vi "Helper SubVI - Get Single-level Coefficients and Reconstructions.vi"(5 "type":enum16{"Apprx", "Detail"}(ring), 6 "synthesis filters":cluster{"lowpass":dbl[], "highpass":dbl[]} {"highpass" format="%.2f"; "lowpass" format="%.2f"}, 7 "level":i32, 8 "error in (no error)":errorcluster, 9 "wavelet":u16(ring) items=["db02"=0, "db03"=1, "db04"=2, "db05"=3, "db06"=4, "db07"=5, "db08"=6, "db09"=7, "db10"=8, "db11"=9, "db12"=10, "db13"=11, "db14"=12, "Haar"=13, "bior1_3"=14, "bior1_5"=15, "bior2_2"=16, "bior2_4"=17, "bior2_6"=18, "bior2_8"=19, "bior3_1"=20, "bior3_3"=21, "bior3_5"=22, "bior3_7"=23, "bior3_9"=24, "bior4_4 (FBI)"=25, "bior5_5"=38, "bior6_8"=39, "coif1"=26, "coif2"=27, "coif3"=28, "coif4"=29, "coif5"=30, "sym2"=31, "sym3"=32, "sym4"=33, "sym5"=34, "sym6"=35, "sym7"=36, "sym8"=37], 10 "Lengths":i32[](array[numeric]), 11 "DWT":dbl[](array[numeric]) format="%.2f") -> (0 "error out":errorcluster, 2 "Reconstruction":dbl[](array[numeric]), 3 "Coeffs":dbl[](array[numeric]) format="%.2f")   [LabVIEW 2023]
doc: "Gets single-level coefficients and returns the reconstructed signal."
uses:
  <vilib>/addons/Wavelet Analysis/discrete wavelet transform.llb/WA Inverse 1D Discrete Wavelet Transform (Array).vi
  <vilib>/addons/_Advanced Signal Processing/NI_AdvSigProcWA.lvlib
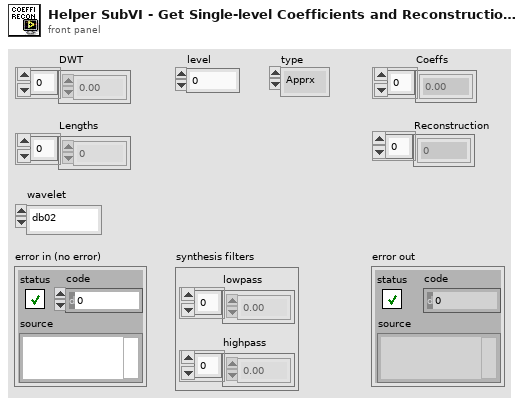
[diagram p1: front panel]
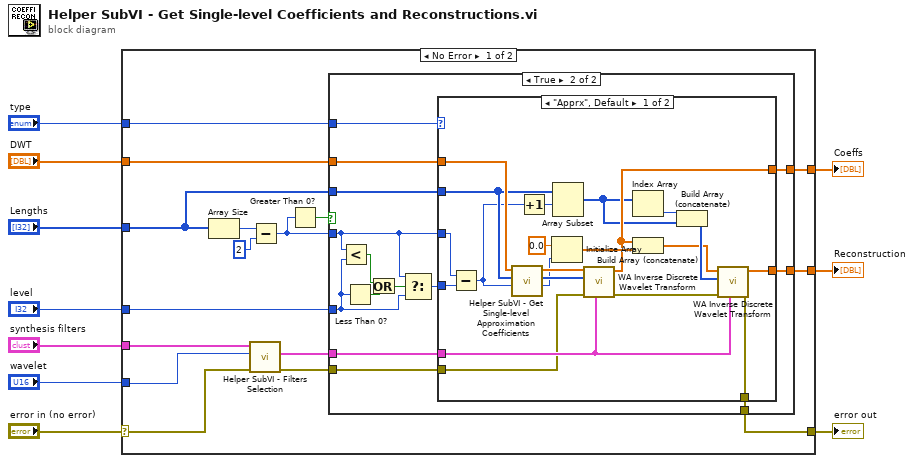
[diagram p0: block diagram]
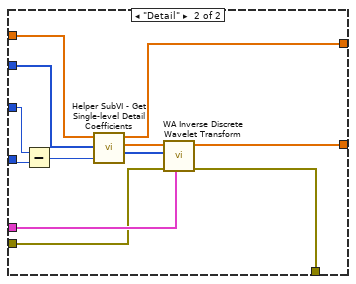
[diagram p3: hidden frame]
diagram:
  n1 = case shown="No Error" "error in (no error)" {
    selector: "error in (no error)" -> [w11 w75]
    tunnel: [w22 w75] -> w9
    tunnel: "DWT" -> [w21 _]
    tunnel: "Lengths" -> [w20 _]
    tunnel: "level" -> [w19 _]
    tunnel: "synthesis filters" -> [w18 _]
    tunnel: "wavelet" -> [w15 _]
    tunnel: [w17 _] -> w3
    tunnel: [w16 _] -> w2
    tunnel: "type" -> [w13 _]
    frame No Error {
      n2 = Array Size(array=w20) -> (size(s)=w26:i32)
      n3 = call "Helper SubVI - Filters Selection.vi"("error in (no error)"=w11, "wavelet"=w15, "filters"=w18) -> ("error out"=w12:errorcluster, "synthesis filters"=w14:cluster{"lowpass":dbl[], "highpass":dbl[]})  [unwired: 6 in, 1 out]
      n4 = Subtract(x=w26, y=2) -> (x-y=w23:i32)
      n5 = Greater Than 0?(x=w23) -> (x > 0?=w24:bool)
      n6 = case shown="True" w24 {
        tunnel: w21 -> [_ w39]
        tunnel: [_ w40] -> w16
        tunnel: w23 -> [_ w32]
        tunnel: w19 -> [_ w31]
        tunnel: w20 -> [_ w41]
        tunnel: w14 -> [_ w38]
        tunnel: [w27 w37] -> w22
        tunnel: [_ w36] -> w17
        tunnel: w13 -> [_ w29]
        tunnel: w12 -> [w27 w28]
        frame False {
        }
        frame True {
          n7 = Less?(x=w32, y=w31) -> (x < y?=w33:bool)
          n8 = Less Than 0?(x=w31) -> (x < 0?=w30:bool)
          n9 = Or(x=w33, y=w30) -> (x .or. y?=w35:bool)
          n10 = Select(t=w32, s=w35, f=w31) -> (s? t:f=w34:i32)
          n11 = case shown="\"Apprx\", Default" w29 {
            tunnel: w39 -> [w60 w74]
            tunnel: w41 -> [w51 w68]
            tunnel: [w52 w73] -> w40
            tunnel: w34 -> [w59 w65]
            tunnel: w38 -> [w56 w71]
            tunnel: [w62 w70] -> w37
            tunnel: [w61 w69] -> w36
            tunnel: w32 -> [w44 w66]
            tunnel: w28 -> [w42 w63]
            frame "Apprx", Default {
              n12 = Subtract(x=w44, y=w59) -> (x-y=w49:i32)
              n13 = call "Helper SubVI - Get Single-level Approximation Coefficients.vi"("index of Lengths"=w49, "Lengths"=w51, "DWT"=w60) -> ("left length"=w55:i32, "Lengths out"=w57:i32[], "DWT 2"=w58:dbl[])  [unwired: 6 in]
              n14 = Increment(x=w49) -> (x+1=w50:i32)
              n15 = Initialize Array(0.0 ("element"), w55) -> (w53:dbl[])
              n16 = Array Subset(array=w51, index=w50) -> (w47:i32[])  [unwired: 1 in]
              n17 = call-poly <vilib>:"WA Inverse Discrete Wavelet Transform.vi"("synthesis filters"=w56, "error in (no error)"=w42, "length"=w57, "DWT coef"=w58) -> ("error out"=w45:errorcluster, "signal"=w52:dbl[])  [unwired: 1 in, 5 out]
              n18 = Index Array(array=w47) -> (element=w48:i32)  [unwired: 1 in]
              n19 = Build Array (concatenate)(w52, w53) -> (w43:dbl[])
              n20 = Build Array (concatenate)(w48, w47) -> (w46:i32[])
              n21 = call-poly <vilib>:"WA Inverse Discrete Wavelet Transform.vi"("synthesis filters"=w56, "error in (no error)"=w45, "length"=w46, "DWT coef"=w43) -> ("error out"=w62:errorcluster, "signal"=w61:dbl[])  [unwired: 1 in, 5 out]
            }
            frame "Detail" {
              n22 = Subtract(x=w66, y=w65) -> (x-y=w64:i32)
              n23 = call "Helper SubVI - Get Single-level Detail Coefficients.vi"("index of Lengths"=w64, "Lengths"=w68, "DWT"=w74) -> ("Lengths out"=w67:i32[], "DWT 2"=w72:dbl[], "Coeffs"=w73:dbl[])  [unwired: 6 in]
              n24 = call-poly <vilib>:"WA Inverse Discrete Wavelet Transform.vi"("synthesis filters"=w71, "error in (no error)"=w63, "length"=w67, "DWT coef"=w72) -> ("error out"=w70:errorcluster, "signal"=w69:dbl[])  [unwired: 1 in, 5 out]
            }
          }
        }
      }
    }
    frame Error {
    }
  }
  "error out" <- w9
  "Coeffs" <- w2
  "Reconstruction" <- w3
